vi "Weather Station UI.vi"() -> ()   [LabVIEW 2014]
doc: "This is the main VI in the Weather Station Project. It contains the user interface for a temperature warning system. Temperature is retrieved every half second; data is logged when a warning has occurred."
uses:
  Supporting Files/Weather Station States.ctl
  Supporting Files/Weather Data.ctl
  Instance           2 26Saved   Weather Station UI .vi
panel:
  out "Warning":string
  in  "Lower Limit":dbl=20.0
  in  "Upper Limit":dbl=30.0
  in  "Stop Button":bool
  out "Temperature History":dbl(graph)
  # "Temperature Ranges (C)"
  # "Freeze"
  # "Heat \nStroke"
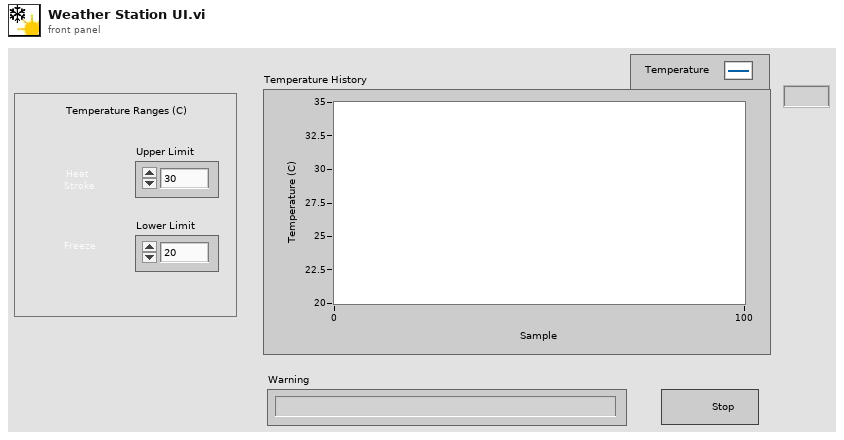
[diagram p1: front panel]
types:
  T1 = enum16{"open", "replace", "create", "open or create", "replace or create", "replace or create with confirmation"}
  T2 = typedef "Weather Data.ctl" = cluster{"Current Temperature":dbl, "Max Temperature":dbl, "Min Temperature":dbl, "Temperature Warning?":bool, "Temperature Warning Text":string}
  T3 = typedef "Weather Station States.ctl" = enum16{"Acquisition", "Analysis", "Data Log", "Time Check"}
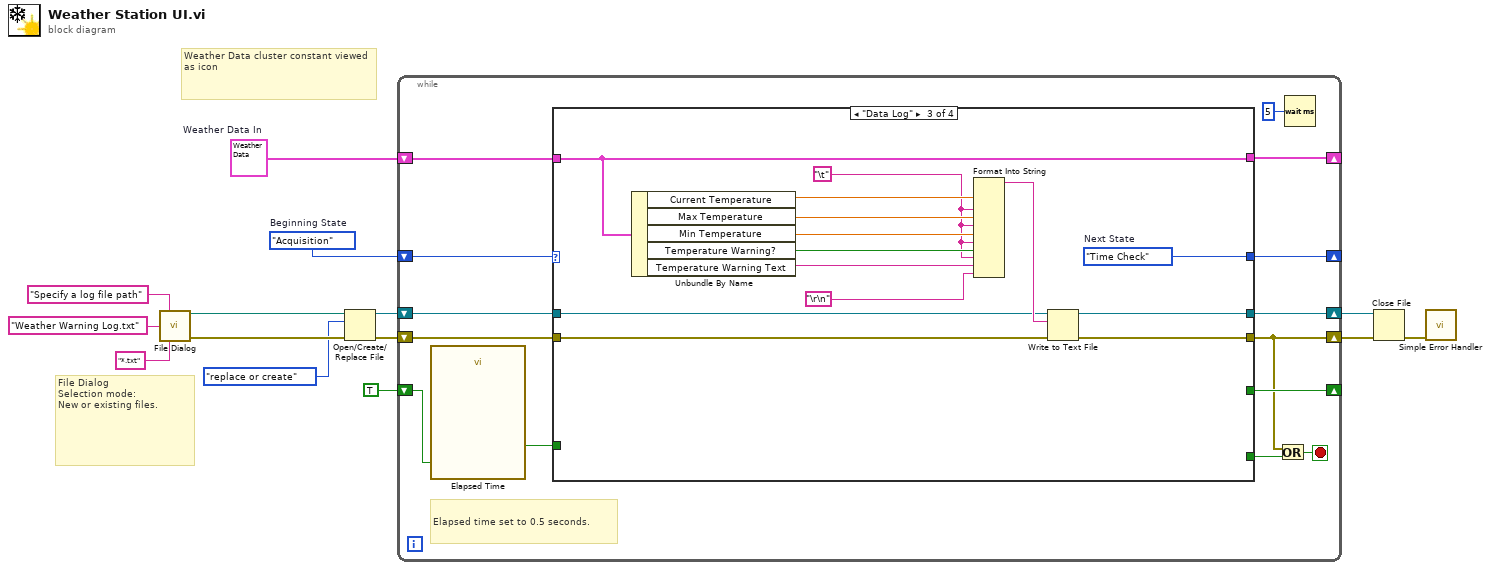
[diagram p0: block diagram]
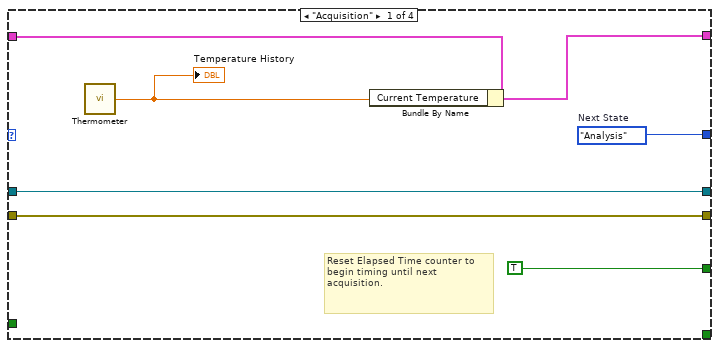
[diagram p2: hidden frame]
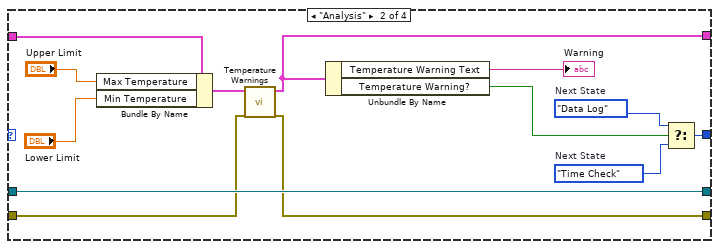
[diagram p3: hidden frame]
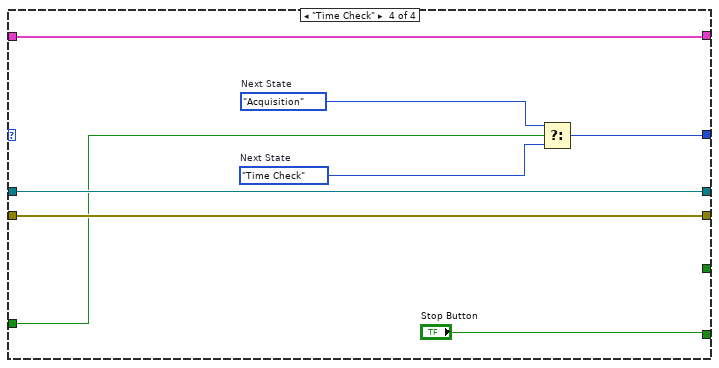
[diagram p4: hidden frame]
diagram:
  w7 = T2 {"Current Temperature"=0.0, "Max Temperature"=0.0, "Min Temperature"=0.0, "Temperature Warning?"=FALSE, "Temperature Warning Text"="No Warning"}  # Weather Data In
  w14 = Weather_Station_States."Acquisition"  # Beginning State
  # "File Dialog\nSelection mode:\nNew or existing files."
  # "Weather Data cluster constant viewed as icon"
  n1 = call "File Dialog"("prompt"="Specify a log file path", "default name"="Weather Warning Log.txt", "pattern (all files)"="*.txt" ("pattern label")) -> ("selected path"=w6:path, "error out"=w3:errorcluster)  [unwired: 9 in, 2 out]
  n2 = Open/Create/Replace File(file path (use dialog)=w6, error in=w3, operation (0:open)=T1."replace or create") -> (refnum out=w9:refnum<file>, error out=w8:errorcluster)  [unwired: 3 in, 1 out]
  n3 = while {
    shift-right: [w27] -> _
    shift-left: w14 -> [w28]
    shift-right: [w15] -> w13
    shift-left: w8 -> [w26]
    shift-right: [w16] -> _
    shift-left: w7 -> [w23]
    shift-right: [w24] -> w12
    shift-left: w9 -> [w22]
    shift-right: [w17] -> _
    shift-left: TRUE ("stop") -> [w19]
    stop <- w25 stop-if-true
    # "Elapsed time set to 0.5 seconds."
    n4 = call "Elapsed Time"("Reset"=w19) -> ("Time has Elapsed"=w18:bool)  [unwired: 11 in, 7 out]
    n5 = case shown="\"Data Log\"" w28 {
      tunnel: [w35 w42 w62 w63] -> w27
      tunnel: [w30 w46 w60 w69] -> w15
      tunnel: w26 -> [w30 w47 w61 w69]
      tunnel: [w34 w48 w59 w70] -> w24
      tunnel: [w31 w41 w51 w68] -> w16
      tunnel: w23 -> [w32 w39 w51 w68]
      tunnel: w22 -> [w34 w48 w57 w70]
      tunnel: [_ _ _ "Stop Button"] -> w21
      tunnel: w18 -> [_ _ _ w64]
      tunnel: [TRUE ("stop") _ _ _] -> w17
      frame "Acquisition" {
        w35 = Weather_Station_States."Analysis"  # Next State
        # "Reset Elapsed Time counter to begin timing until next acquisition."
        n6 = call "Thermometer.vi"() -> ("Temperature"=w29:dbl)  [unwired: 1 in]
        "Temperature History" <- w29
        n7 = Bundle By Name(cluster=w32, "Current Temperature"=w29) -> (w31:T2)
      }
      frame "Analysis" {
        w44 = Weather_Station_States."Data Log"  # Next State
        w43 = Weather_Station_States."Time Check"  # Next State
        n8 = Bundle By Name(cluster=w39, "Max Temperature"="Upper Limit", "Min Temperature"="Lower Limit") -> (w38:T2)
        n9 = call "Temperature Warnings.vi"("Error In"=w47, "Weather Data In"=w38) -> ("Error Out"=w46:errorcluster, "Weather Data Out"=w41:T2)  [unwired: 8 in]
        n10 = Unbundle By Name(w41) -> ("Temperature Warning Text"=→"Warning":string, "Temperature Warning?"=w45:bool)
        n11 = Select(t=w44, s=w45, f=w43) -> (s? t:f=w42:T3)
      }
      frame "Data Log" {
        w62 = Weather_Station_States."Time Check"  # Next State
        w50 = "\t"
        n12 = Unbundle By Name(w51) -> ("Current Temperature"=w56:dbl, "Max Temperature"=w55:dbl, "Min Temperature"=w54:dbl, "Temperature Warning?"=w53:bool, "Temperature Warning Text"=w49:string)
        n13 = Format Into String(w56, w50, w55, w50, w54, w50, w53, w50, w49, "\r\n") -> (resulting string=w58:string)  [unwired: 3 in, 1 out]
        n14 = Write to Text File(file (use dialog)=w57, text=w58, error in=w61) -> (refnum out=w59:refnum<file>, error out=w60:errorcluster)  [unwired: 1 in, 1 out]
      }
      frame "Time Check" {
        w66 = Weather_Station_States."Time Check"  # Next State
        w65 = Weather_Station_States."Acquisition"  # Next State
        n15 = Select(t=w65, s=w64, f=w66) -> (s? t:f=w63:T3)
      }
    }
    n16 = Or(x=w15, y=w21) -> (x .or. y?=w25:bool)
    n17 = Wait (ms)(milliseconds to wait=u32 5 ("y")) -> ()  [unwired: 1 out]
  }
  n18 = Close File(refnum=w12, error in=w13) -> (error out=w11:errorcluster)  [unwired: 1 out]
  n19 = call <vilib>:"Simple Error Handler.vi"("error in (no error)"=w11) -> ()  [unwired: 4 in, 5 out]
